vi "Unit3.vi"   [LabVIEW 2021]
uses:
  GUI_Def.ctl
types:
  T1 = enum16{"open", "replace", "create", "open or create", "replace or create", "replace or create with confirmation"}
  T2 = typedef "GUI_Def.ctl" = cluster{"Monitor MSG":string, "Request Read":bool, "Time Stamp":timestamp, "CV":cluster{"Background":bool, "BackgroundArray":cluster{timestamp, i32}[], "SetPointArray":cluster{timestamp, i32}[]}, "Normal":cluster{"Collecting":bool}, "Getting Mode":enum16{"Off", "Normal", "CV"}}
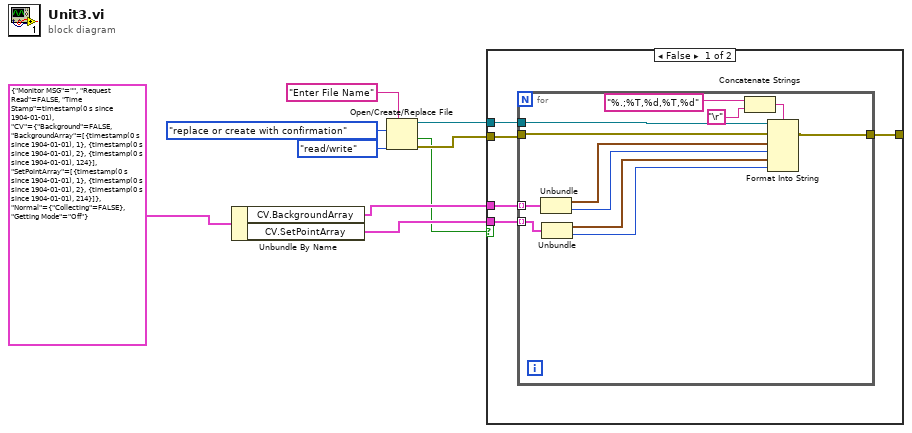
[diagram p0: block diagram]
diagram:
  n1 = Unbundle By Name(T2 {"Monitor MSG"="", "Request Read"=FALSE, "Time Stamp"=timestamp(0 s since 1904-01-01), "CV"={"Background"=FALSE, "BackgroundArray"=[{timestamp(0 s since 1904-01-01), 1}, {timestamp(0 s since 1904-01-01), 2}, {timestamp(0 s since 1904-01-01), 124}], "SetPointArray"=[{timestamp(0 s since 1904-01-01), 1}, {timestamp(0 s since 1904-01-01), 2}, {timestamp(0 s since 1904-01-01), 214}]}, "Normal"={"Collecting"=FALSE}, "Getting Mode"=enum."Off"}) -> ("CV.BackgroundArray"=w8:cluster{timestamp, i32}[], "CV.SetPointArray"=w7:cluster{timestamp, i32}[])
  n2 = Open/Create/Replace File(prompt="Enter File Name", operation (0:open)=T1."replace or create with confirmation", access (0:read/write)=enum16{"read/write", "read-only", "write-only"}."read/write") -> (refnum out=w5:refnum<file>, cancelled=w1:bool, error out=w6:errorcluster)  [unwired: 3 in]
  n3 = case shown="False" w1 {
    tunnel: w8 -> [w14 _]
    tunnel: w7 -> [w13 _]
    tunnel: w6 -> [w12 w27]
    tunnel: w5 -> [w11 _]
    tunnel: [w10 w27] -> _
    frame False {
      n4 = for {
        tunnel: w14 -> [w26] mode=indexing
        tunnel: w13 -> [w25] mode=indexing
        tunnel: w11 -> [w24]
        tunnel: w12 -> [w23]
        tunnel: [w15] -> w10
        n5 = Unbundle(w26) -> (w22:timestamp, w21:i32)
        n6 = Unbundle(w25) -> (w20:timestamp, w19:i32)
        n7 = Concatenate Strings("%.;%T,%d,%T,%d" ("format string"), "\r") -> (w16:string)
        n8 = Format Into String(format string=w16, initial string=w24, error in=w23, w22, w21, w20, w19) -> (error out=w15:errorcluster)  [unwired: 1 out]
      }
    }
    frame True {
    }
  }
